vi "3способа.vi"() -> ()   [LabVIEW 2017]
panel:
  out "Полиморфизм":dbl[](array[numeric])
  out "Регистр сдвига":dbl[](array[numeric])
  out "Знаечния логарифма":dbl[](array[numeric])
  out "Array - Автоиндексация":dbl[](array[numeric])
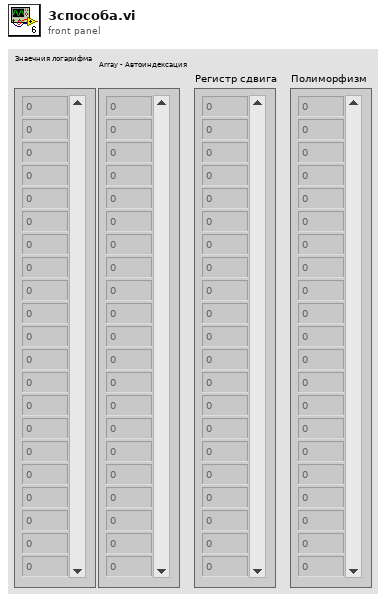
[diagram p1: front panel]
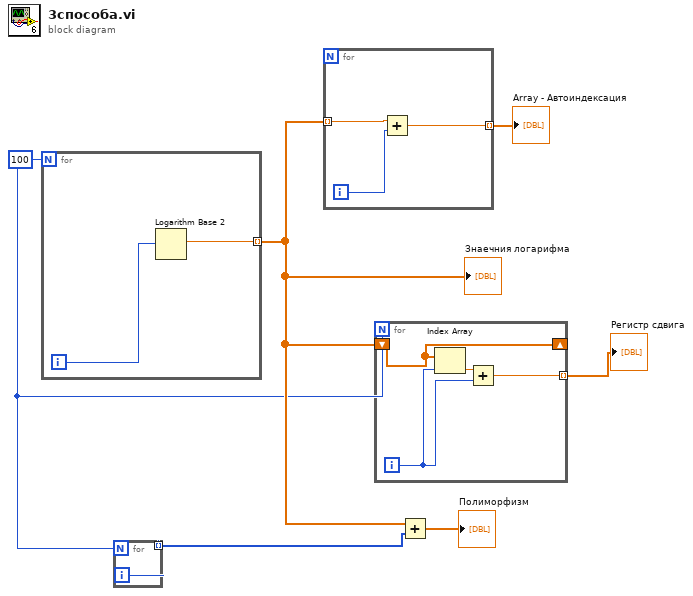
[diagram p0: block diagram]
diagram:
  w3 = 100
  n1 = for {
    N: w3 -> [_]
    tunnel: [w7] -> w4 mode=indexing
    i -> [w8]
    n2 = Logarithm Base 2(1:w8) -> (0:w7:dbl)
  }
  "Знаечния логарифма" <- w4
  n3 = for {
    N: w3 -> [_]
    tunnel: [w9] -> w2 mode=indexing
    i -> [w9]
  }
  n4 = for {
    tunnel: w4 -> [w12] mode=indexing
    tunnel: [w10] -> w6 mode=indexing
    i -> [w11]
    n5 = Add(x=w12, y=w11) -> (x+y=w10:dbl)
  }
  "Array - Автоиндексация" <- w6
  n6 = for {
    N: w3 -> [_]
    shift-right: [w13] -> _
    shift-left: w4 -> [w13]
    tunnel: [w14] -> w5 mode=indexing
    i -> [w16]
    n7 = Index Array(array=w13, index=w16) -> (element=w15:dbl)
    n8 = Add(x=w15, y=w16) -> (x+y=w14:dbl)
  }
  "Регистр сдвига" <- w5
  n9 = Add(x=w4, y=w2) -> (x+y=→"Полиморфизм":dbl[])
